vi "hd.vi"() -> ()   [LabVIEW 2023]
uses:
  <vilib>/DAQmx/write.llb/DAQmx Write (Digital Bool 1Line 1Point).vi
  <vilib>/DAQmx/create/channels.llb/DAQmx Create Channel (DO-Digital Output).vi
  <vilib>/DAQmx/miscellaneous.llb/DAQmx Fill In Error Info.vi
panel:
  in  "Boolean":bool
  in  "stop":bool
  in  "lines 2":tag
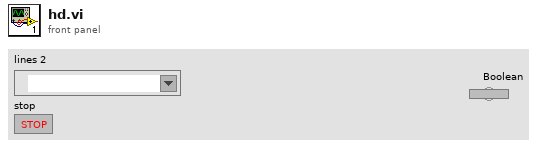
[diagram p1: front panel]
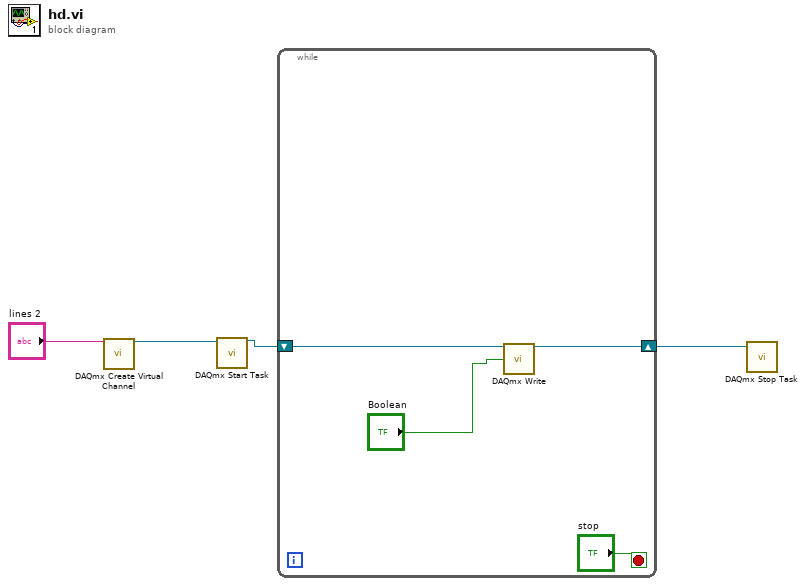
[diagram p0: block diagram]
diagram:
  n1 = call-poly <vilib>:"DAQmx Create Virtual Channel.vi"("lines"="lines 2") -> ("task out"=w3:refnum<k21>)  [unwired: 13 in, 1 out]
  n2 = call <vilib>:"DAQmx Start Task.vi"("task/channels in"=w3) -> ("task out"=w2:refnum<k21>)  [unwired: 13 in, 1 out]
  n3 = while {
    shift-right: [w7] -> w1
    shift-left: w2 -> [w8]
    stop <- "stop" stop-if-true
    n4 = call-poly <vilib>:"DAQmx Write.vi"("task/channels in"=w8, "data"="Boolean") -> ("task out"=w7:refnum<k21>)  [unwired: 11 in, 2 out]
  }
  n5 = call <vilib>:"DAQmx Stop Task.vi"("task/channels in"=w1) -> ()  [unwired: 13 in, 2 out]
